vi "Example_Download_NETHTTPClient.vi"() -> ()   [LabVIEW 2018, in "HttpExamples.lvlib"]
uses:
  <vilib>/Utility/sysdir.llb/System Directory Type.ctl
  Types/ScaledValue_ring.ctl
  c69d9733-6763-4a55-8803-753516d85c26.vi
  7c1dfb00-8e8e-4235-b19c-ed0f93283bd3.vi
  LabVIEWHTTPClient_NET/Accessors/Write RequestHeaderContentFirst.vi
  Types/method_enum.ctl
  Types/DownloadStats_Cluster.ctl
  HttpExamples.lvlib
  LabVIEWHTTPClient_NET/LabVIEWHTTPClient_NET.lvclass
  LabVIEWHTTPClient_NET.lvlib
  HttpResponseMessage/HttpResponseMessage.lvclass
  HttpContent/HttpContent.lvclass
  HttpDownloadTask/HttpDownloadTask.lvclass
panel:
  out "Canceled":bool
  in  "Abort":bool
  out "Progress":dbl(slide) scale=0.0..1.0
  out "Status":string
  out "IsCompleted":bool
  out "error out":errorcluster
  in  "URL":string="https://github.com/git-for-windows/git/releases/download/v2.30.0.windows.2/Git-2.30.0.2-64-bit.exe"
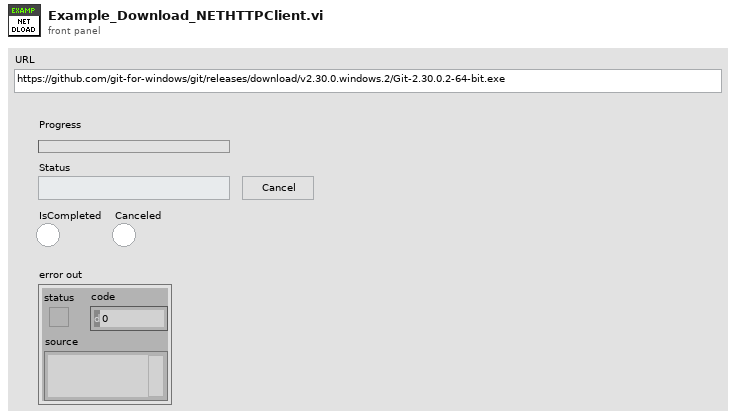
[diagram p1: front panel]
types:
  T1 = typedef "System Directory Type.ctl" = i32
  T2 = typedef "LabVIEWHTTPClient_NET.lvlib/DownloadStats_Cluster.ctl" = cluster{"PositionCurrent":dbl, "PositionPrev":dbl, "TimeCurrent":timestamp, "TimePrev":timestamp, "TimeTotal":dbl, "PositionTotal":dbl, "TimeArray":dbl[], "PositionDifArray":dbl[], "CurrentRate":dbl, "RunningRate_10":dbl, "RunningRate":dbl, "Length":dbl}
  T3 = typedef "LabVIEWHTTPClient_NET.lvlib/method_enum.ctl" = enum16{"GET", "PUT", "POST", "DELETE", "HEAD", "TRACE", "SEND"}
  T4 = typedef "LabVIEWHTTPClient_NET.lvlib/ScaledValue_ring.ctl" = u64
  T5 = typedef "LabVIEWHTTPClient_NET.lvlib/HttpDownloadTask.lvclass/DownloadTask_ref.ctl" = refnum<data-value>
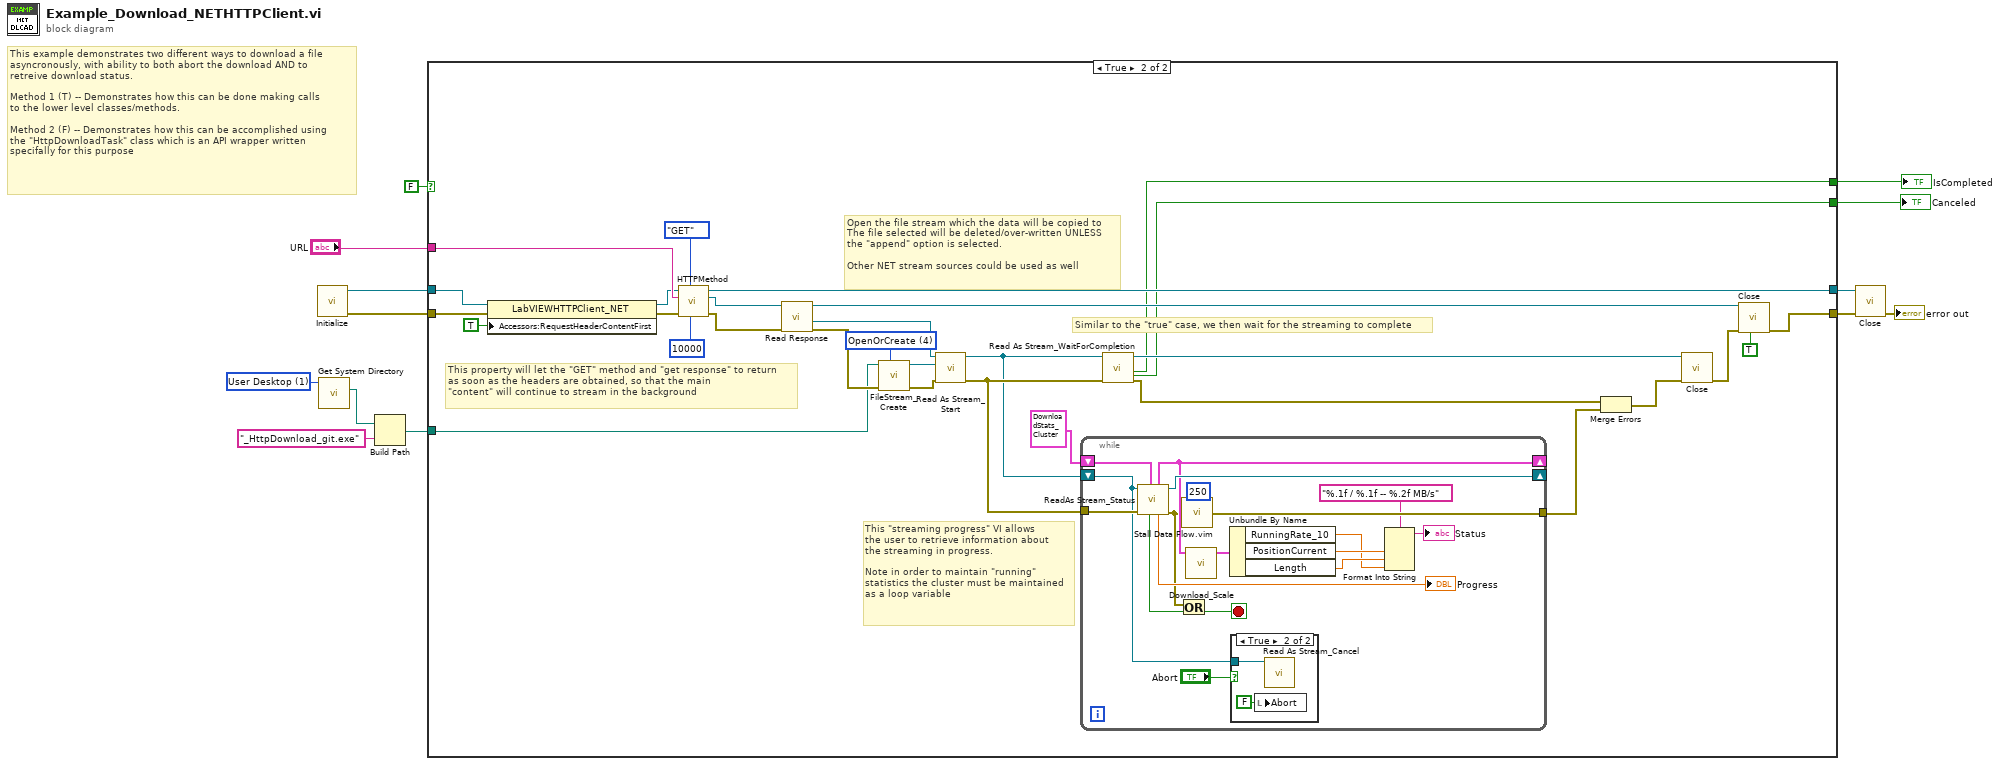
[diagram p0: block diagram]
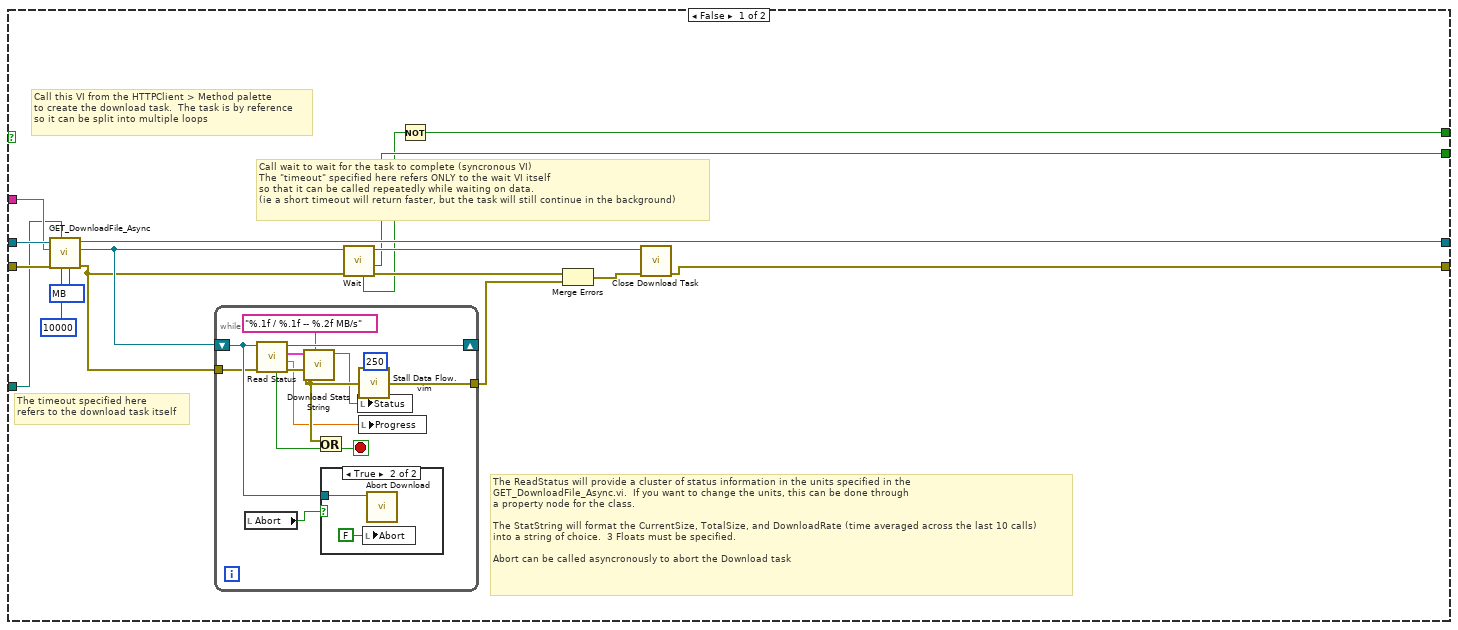
[diagram p2: hidden frame]
diagram:
  w5 = T1 1 items=["User Home"=0, "User Desktop"=1, "User Documents"=2, "User Application Data"=3, "User Preferences"=4, "User Temporary"=5, "Public Documents"=6, "Public Application Data"=7, "Public Preferences"=8, "Public Cache"=13, "System Core Libraries"=9, "System Installed Libraries"=10, "Application Files"=11, "Boot Volume Root"=12] ("system directory type")
  # "This example demonstrates two different ways to download a file\nasyncronously, with ability to both abort the download AND to\nretreive download status.\n\nMethod 1 (T) -- Demonstrates how this can be done making calls\nto the lower level classes/methods.\n\nMethod 2 (F) -- Demonstrates how this can be accomplished using\nthe \"HttpDownloadTask\" class which is an API wrapper written\nspecifally for this purpose"
  n1 = call "Initialize.vi"() -> ("error out"=w6:errorcluster, "HTTP Client Out"=w7:refnum<class "LabVIEWHTTPClient_NET.lvclass">)  [unwired: 10 in]
  n2 = call <vilib>:"Get System Directory.vi"("system directory type"=w5) -> ("system directory"=w4:path)  [unwired: 10 in]
  n3 = Build Path(base path=w4, name or relative path="_HttpDownload_git.exe") -> (appended path=w2:path)
  n4 = case shown="True" FALSE {
    tunnel: [w25 w75] -> w12
    tunnel: "URL" -> [w28 w73]
    tunnel: [w19 w69] -> w10
    tunnel: [w16 w58] -> w9
    tunnel: [w18 w50] -> w8
    tunnel: w7 -> [w29 w48]
    tunnel: w6 -> [w30 w47]
    tunnel: w2 -> [w27 w46]
    frame False {
      w14 = T4 1000000 items=["Bytes"=1, "KB"=1000, "MB"=1000000, "GB"=1000000000] ("Prefered Stat Scale [MB]")
      # "The ReadStatus will provide a cluster of status information in the units specified in the \nGET_DownloadFile_Async.vi.  If you want to change the units, this can be done through\na property node for the class.\n\nThe StatString will format the CurrentSize, TotalSize, and DownloadRate (time averaged across the last 10 calls)\ninto a string of choice.  3 Floats must be specified.\n\nAbort can be called asyncronously to abort the Download task"
      # "Call wait to wait for the task to complete (syncronous VI)\nThe \"timeout\" specified here refers ONLY to the wait VI itself\nso that it can be called repeatedly while waiting on data.\n(ie a short timeout will return faster, but the task will still continue in the background)"
      # "The timeout specified here\nrefers to the download task itself"
      # "Call this VI from the HTTPClient > Method palette\nto create the download task.  The task is by reference\nso it can be split into multiple loops"
      n5 = call "GET_DownloadFile_Async.vi"("Prefered Stat Scale [MB]"=w14, "Timeout_ms (10000)"=10000, "TargetFilePath"=w27, "error in (no error)"=w30, "URL"=w28, "LabVIEWHTTPClient_NET in"=w29) -> ("error out"=w23:errorcluster, "DownloadTask Ref"=w24:T5, "LabVIEWHTTPClient_NET out"=w25:refnum<class "LabVIEWHTTPClient_NET.lvclass">)  [unwired: 3 in]
      n6 = while {
        shift-right: [w38] -> _
        shift-left: w24 -> [w39]
        tunnel: [w43] -> w21
        tunnel: w23 -> [w36]
        stop <- w41 stop-if-true
        n7 = local read "Abort"() -> (w40:bool)
        n8 = call "Read Status.vi"("error in (no error)"=w36, "HttpDownloadTask in"=w39) -> ("error out"=w37:errorcluster, "Progress"=w32:dbl, "RunningStats"=w35:T2, "HttpDownloadTask out"=w38:T5, "Done or Error"=w31:bool)  [unwired: 5 in]
        n9 = call "Download Stats String.vi"("Format String (3 floats)"="%.1f / %.1f -- %.2f MB/s" ("format string"), "Status Cluster"=w35) -> ("Status String"=w33:string)  [unwired: 8 in, 1 out]
        n10 = Or(x=w37, y=w31) -> (x .or. y?=w41:bool)
        n11 = case shown="True" w40 {
          tunnel: w39 -> [_ w44]
          frame False {
          }
          frame True {
            n12 = local write "Abort"(FALSE ("Abort")) -> ()
            n13 = call "Abort Download.vi"("HttpDownloadTask in"=w44) -> ()  [unwired: 9 in, 2 out]
          }
        }
        n14 = local write "Status"(w33) -> ()
        n15 = call "Stall Data Flow.vim"("value in"=w37, "milliseconds to wait"=u32 250) -> ("value out"=w43:errorcluster)  [unwired: 1 out]
        n16 = local write "Progress"(w32) -> ()
      }
      n17 = call "Wait.vi"("error in (no error)"=w23, "HttpDownloadTask in"=w24) -> ("error out"=w22:errorcluster, "Canceled"=w18:bool, "HttpDownloadTask out"=w26:T5, "Wait Timed out"=w17:bool)  [unwired: 6 in]
      n18 = Not(x=w17) -> (.not. x?=w16:bool)
      n19 = Merge Errors(w22, w21) -> (w20:errorcluster)
      n20 = call "Close Download Task.vi"("error in (no error)"=w20, "HttpDownloadTask in"=w26) -> ("error out"=w19:errorcluster)  [unwired: 9 in]
    }
    frame True {
      w56 = 4 items=["CreateNew"=1, "Create"=2, "Open"=3, "OpenOrCreate"=4, "Truncate"=5, "Append"=6] ("mode [CreateNew]")
      # "This \"streaming progress\" VI allows\nthe user to retrieve information about\nthe streaming in progress.\n\nNote in order to maintain \"running\" \nstatistics the cluster must be maintained\nas a loop variable"
      # "Similar to the \"true\" case, we then wait for the streaming to complete"
      # "Open the file stream which the data will be copied to\nThe file selected will be deleted/over-written UNLESS\nthe \"append\" option is selected.\n\nOther NET stream sources could be used as well"
      # "This property will let the \"GET\" method and \"get response\" to return\nas soon as the headers are obtained, so that the main\n\"content\" will continue to stream in the background"
      n21 = property class="LabVIEWHTTPClient_NET"(reference=w48, error in=w47, "Accessors:RequestHeaderContentFirst"=TRUE ("RequestHeaderContentFirst")) -> (reference out=w66:refnum<class "LabVIEWHTTPClient_NET.lvclass">, error out=w67:errorcluster)
      n22 = call "HTTPMethod.vi"("Timeout_ms (10000)"=10000, "Method"=method_enum."GET", "error in (no error)"=w67, "URL"=w73, "LabVIEWHTTPClient_NET in"=w66) -> ("error out"=w63:errorcluster, "HttpResponseMessage out"=w49:refnum<class "HttpResponseMessage.lvclass">, "LabVIEWHTTPClient_NET out"=w75:refnum<class "LabVIEWHTTPClient_NET.lvclass">)  [unwired: 4 in]
      n23 = call "Read Response.vi"("error in (no error)"=w63, "HttpResponseMessage in"=w49) -> ("error out"=w62:errorcluster, "HttpContent out"=w61:refnum<class "HttpContent.lvclass">, "HttpResponseMessage out"=w72:refnum<class "HttpResponseMessage.lvclass">)  [unwired: 3 in, 4 out]
      n24 = call "FileStream_Create.vi"("mode [OpenOrCreate]"=w56, "error in (no error)"=w62, "FilePath"=w46) -> ("error out"=w60:errorcluster, "FileStream"=w55:refnum<k24>)  [unwired: 7 in]
      n25 = call "Read As Stream_Start.vi"("error in (no error)"=w60, "DestinationStream"=w55, "HttpContent in"=w61) -> ("error out"=w54:errorcluster, "HttpContent out"=w53:refnum<class "HttpContent.lvclass">)  [unwired: 7 in]
      n26 = while {
        shift-right: [w92] -> _
        shift-left: w53 -> [w78]
        tunnel: w54 -> [w93]
        tunnel: [w91] -> w52
        shift-right: [w87] -> _
        shift-left: T2 {"PositionCurrent"=0.0, "PositionPrev"=0.0, "TimeCurrent"=timestamp(0 s since 1904-01-01), "TimePrev"=timestamp(0 s since 1904-01-01), "TimeTotal"=0.0, "PositionTotal"=0.0, "TimeArray"=[], "PositionDifArray"=[], "CurrentRate"=0.0, "RunningRate_10"=0.0, "RunningRate"=0.0, "Length"=0.0} ("RunningStats Out") -> [w88]
        stop <- w77 stop-if-true
        n27 = call "ReadAs Stream_Status.vi"("DownloadStats In"=w88, "error in (no error)"=w93, "HttpContent in"=w78) -> ("error out"=w76:errorcluster, "HttpContent out"=w92:refnum<class "HttpContent.lvclass">, "Progress"=→"Progress":dbl, "RunningStats Out"=w87:T2, "Done or Error"=w89:bool)  [unwired: 2 in, 2 out]
        n28 = Or(x=w76, y=w89) -> (x .or. y?=w77:bool)
        n29 = call "Stall Data Flow.vim"("value in"=w76, "milliseconds to wait"=u32 250) -> ("value out"=w91:errorcluster)  [unwired: 1 out]
        n30 = call "Download_Scale.vi"("DownloadStats In"=w87) -> ("RunningStats"=w86:T2)  [unwired: 10 in]
        n31 = Unbundle By Name(w86) -> ("RunningRate_10"=w83:dbl, "PositionCurrent"=w85:dbl, "Length"=w84:dbl)
        n32 = case shown="True" "Abort" {
          tunnel: w78 -> [_ w95]
          frame False {
          }
          frame True {
            n33 = local write "Abort"(FALSE ("Abort")) -> ()
            n34 = call "Read As Stream_Cancel.vi"("HttpContent in"=w95) -> ()  [unwired: 9 in, 2 out]
          }
        }
        n35 = Format Into String(format string="%.1f / %.1f -- %.2f MB/s", w85, w84, w83) -> (resulting string=→"Status":string)  [unwired: 2 in, 1 out]
      }
      n36 = call "Read As Stream_WaitForCompletion.vi"("error in (no error)"=w54, "HttpContent in"=w53) -> ("error out"=w57:errorcluster, "IsCompleted"=w58:bool, "HttpContent out"=w59:refnum<class "HttpContent.lvclass">, "Canceled"=w50:bool)  [unwired: 6 in]
      n37 = Merge Errors(w57, w52) -> (w68:errorcluster)
      n38 = call "Close.vi"("error in (no error)"=w68, "HttpContent in"=w59) -> ("error out"=w70:errorcluster)  [unwired: 9 in]
      n39 = call "Close.vi"("CloseHeaders"=TRUE, "error in (no error)"=w70, "HttpResponseMessage in"=w72) -> ("error out"=w69:errorcluster)  [unwired: 8 in]
    }
  }
  "IsCompleted" <- w9
  "Canceled" <- w8
  n40 = call "Close.vi"("Error In"=w10, "LabVIEWHTTPClient_NET in"=w12) -> ("Error Out"=→"error out":errorcluster)  [unwired: 9 in]
